vi "输入数据解析.vi"(0 "单个参数补充":dbl, 1 "从板号":dbl=1.0, 2 "主板二维码":string="BNET01", 3 "从板二维码":string="BNET01", 5 "主板引用":refnum<vi>, 7 "从板引用":refnum<vi>, 9 "主板选项":string="三级故障阀值", 11 "枚举":enum16{"主板", "从板"}(ring), 12 "快换":bool caption="快换写入") -> (4 "输出数组":dbl[][](array[numeric]), 6 "数组长度":dbl[](array[numeric]), 8 "循环次数":i32, 10 "命令":u32, 14 "名称":string[](array[string]), 15 "命令序号":u32[](array[numeric]))   [LabVIEW 2013] (continued)
                n5736 = property class="Tbl (严格)"(reference=w15118) -> ("Value"=w15116:string[][])  [unwired: 1 in, 2 out]
                n5737 = Index Array(array=w15116, index (col)=1 ("禁用的索引 (列)")) -> (element=w15120:string[])  [unwired: 1 in]
                n5738 = Array Subset(array=w15120, index=2 ("索引"), length=20.0 ("y")) -> (w15121:string[])
                n5739 = Fract/Exp String To Number(string=w15121) -> (number=w15113:dbl[])  [unwired: 4 out]
                n5740 = for {
                  N: 10 -> [_]
                  tunnel: w15113 -> [w15133]
                  tunnel: [w15124] -> w15111 mode=indexing
                  i -> [w15135]
                  w15128 = 4 ("索引")
                  n5741 = Multiply(x=w15135, y=2) -> (x*y=w15132:i32)
                  n5742 = Increment(x=w15132) -> (x+1=w15131:i32)
                  n5743 = Index Array(array=w15133, index #1=w15132, index #2=w15131) -> (element #1=w15130:dbl, element #2=w15129:dbl)
                  n5744 = call "二进制解析-8.6.vi"("索引"=w15128, "数值"=w15130) -> ("低位子数组"=w15127:i32[])  [unwired: 1 in, 2 out]
                  n5745 = call "二进制解析-8.6.vi"("索引"=w15128, "数值"=w15129) -> ("低位子数组"=w15126:i32[])  [unwired: 1 in, 2 out]
                  n5746 = Insert Into Array(array=w15127, new element=w15126) -> (w15125:i32[])  [unwired: 1 in]
                  n5747 = call "数值二进制转十进制-8.6.vi"("子数组"=w15125) -> ("十进制数值"=w15124:i32)  [unwired: 4 in]
                }
              }
            }
          }
        }
        frame "温度个数" {
          n5748 = for {
            N: 1 -> [_]
            tunnel: [w15147] -> w15141 mode=indexing
            tunnel: [w15146] -> w15140 mode=indexing
            tunnel: [w15145] -> w15139 mode=indexing
            tunnel: w15138 -> [w15144]
            i -> [w15148]
            n5749 = case shown="0, 默认" w15148 {
              tunnel: w15144 -> [w15156]
              tunnel: [w15152] -> w15147
              tunnel: [4.0 ("y")] -> w15146
              tunnel: [4 ("命令序号")] -> w15145
              frame 0, Default {
                n5750 = Unbundle By Name(w15156) -> ("项目信息 2"=w15157:refnum<vi>)
                n5751 = property class="Tbl (严格)"(reference=w15157) -> ("Value"=w15155:string[][])  [unwired: 1 in, 2 out]
                n5752 = Index Array(array=w15155, index (col)=1 ("禁用的索引 (列)")) -> (element=w15159:string[])  [unwired: 1 in]
                n5753 = Array Subset(array=w15159, index=1 ("索引"), length=1.0 ("y")) -> (w15160:string[])
                n5754 = Fract/Exp String To Number(string=w15160) -> (number=w15153:dbl[])  [unwired: 4 out]
                n5755 = for {
                  N: 1 -> [_]
                  tunnel: w15153 -> [w15171] mode=indexing
                  shift-right: [w15166] -> w15152
                  shift-left: dbl[] [] -> [w15165]
                  n5756 = Quotient & Remainder(x=w15171, y=256.0) -> (x-y*floor(x/y)=w15168:dbl, floor(x/y)=w15169:dbl)
                  n5757 = Build Array(w15169, w15168, 0.0 ("元素"), 1.0 ("元素")) -> (w15167:dbl[])
                  n5758 = Insert Into Array(array=w15165, new element=w15167) -> (w15166:dbl[])  [unwired: 1 in]
                }
              }
            }
          }
        }
        frame "加热控制参数" {
          n5759 = for {
            N: 1 -> [_]
            tunnel: w15178 -> [w15182]
            tunnel: [w15185] -> w15177 mode=indexing
            tunnel: [w15184] -> w15176 mode=indexing
            tunnel: [w15183] -> w15175 mode=indexing
            tunnel: w15174 -> [w15181]
            i -> [w15186]
            n5760 = case shown="0, 默认" w15186 {
              tunnel: w15181 -> [w15206 w15212 w15253 w15297 w15341]
              tunnel: w15182 -> [_ w15216 w15257 w15301 w15346]
              tunnel: [w15192 w15217 w15262 w15306 w15345] -> w15185
              tunnel: [7.0 w15218 w15263 w15307 w15344] -> w15184
              tunnel: [u32 5 ("命令序号") u32 2 ("命令序号") u32 3 ("命令序号") u32 4 ("命令序号") u32 1 ("命令序号")] -> w15183
              frame 0, Default {
                n5761 = Unbundle By Name(w15206) -> ("加热控制参数"=w15207:refnum<vi>)
                n5762 = property class="Clust (严格)"(reference=w15207) -> ("Value"=w15205:T5)  [unwired: 1 in, 2 out]
                n5763 = Unbundle(w15205) -> ("风机开启温度"=w15200:dbl, "风机关闭温度"=w15199:dbl, "加热开启温度"=w15196:dbl, "加热关闭温度"=w15195:dbl, "风机开启温差"=w15191:dbl, "风机关闭温差"=w15190:dbl, "加热关闭温差"=w15187:dbl)
                n5764 = call "输入分辨率计算-EV05.vi"("1字节?"=TRUE, "数值 2"=w15195, "数值"=w15196, "偏移量"=-40.0, "分辨率"=1.0) -> ("高字节 2"=w15188:dbl, "高字节1"=w15189:dbl)  [unwired: 5 out]
                n5765 = call "输入分辨率计算-EV05.vi"("1字节?"=TRUE, "数值 2"=w15199, "数值"=w15200, "偏移量"=-40.0, "分辨率"=1.0) -> ("高字节 2"=w15194:dbl, "高字节1"=w15193:dbl)  [unwired: 5 out]
                n5766 = Build Array(w15193, w15194, w15191, w15190, w15189, w15188, w15187) -> (w15192:dbl[])
              }
              frame 1 {
                # "电压起始值"
                n5767 = Unbundle By Name(w15212) -> ("项目信息 2"=w15211:refnum<vi>)
                n5768 = property class="Tbl (严格)"(reference=w15211) -> ("Value"=w15210:string[][])  [unwired: 1 in, 2 out]
                n5769 = Index Array(array=w15210, index (col)=1 ("禁用的索引 (列)")) -> (element=w15224:string[])  [unwired: 1 in]
                n5770 = Multiply(x=w15216, y=6.0) -> (x*y=w15220:dbl)
                n5771 = Divide(x=w15216, y=2.0) -> (x/y=w15214:dbl)
                n5772 = Multiply(x=w15216, y=1.5) -> (x*y=w15227:dbl)
                n5773 = Array Subset(array=w15224, index=w15220, length=w15216) -> (w15222:string[])
                n5774 = Round Toward +Infinity(x=w15214) -> (ceil(x): smallest int >= x=w15213:dbl)
                n5775 = Round Toward +Infinity(x=w15227) -> (ceil(x): smallest int >= x=w15218:dbl)
                n5776 = Fract/Exp String To Number(string=w15222) -> (number=w15225:dbl[])  [unwired: 4 out]
                n5777 = for {
                  N: w15213 -> [_]
                  tunnel: w15225 -> [w15251]
                  tunnel: [w15229] -> w15228 mode=indexing
                  i -> [w15250]
                  w15241 = 256.0 ("y")
                  n5778 = Multiply(x=w15250, y=2) -> (x*y=w15248:i32)
                  n5779 = Increment(x=w15248) -> (x+1=w15247:i32)
                  n5780 = Index Array(array=w15251, index #1=w15248, index #2=w15247) -> (element #1=w15242:dbl)  [unwired: 1 out]
                  n5781 = Quotient & Remainder(x=w15242, y=w15241) -> (x-y*floor(x/y)=w15230:dbl, floor(x/y)=w15238:dbl)
                  n5782 = Quotient & Remainder(x=w15242, y=w15241) -> (x-y*floor(x/y)=w15239:dbl, floor(x/y)=w15240:dbl)
                  n5783 = call "二进制解析-8.6.vi"("索引"=4, "数值"=w15238) -> ("低位子数组"=w15234:i32[])  [unwired: 3 out]
                  n5784 = call "二进制解析-8.6.vi"("索引"=4, "数值"=w15240) -> ("低位子数组"=w15237:i32[])  [unwired: 3 out]
                  n5785 = call "二进制解析-8.6.vi"("索引"=4, "数值"=w15239) -> ("低位子数组"=w15235:i32[], "高位子数组"=w15236:i32[])  [unwired: 2 out]
                  n5786 = Insert Into Array(array=w15237, new element=w15236) -> (w15244:i32[])  [unwired: 1 in]
                  n5787 = Insert Into Array(array=w15235, new element=w15234) -> (w15233:i32[])  [unwired: 1 in]
                  n5788 = call "数值二进制转十进制-8.6.vi"("子数组"=w15233) -> ("十进制数值"=w15231:i32)  [unwired: 4 out]
                  n5789 = call "数值二进制转十进制-8.6.vi"("子数组"=w15244) -> ("十进制数值"=w15232:i32)  [unwired: 4 out]
                  n5790 = Build Array(w15232, w15231, w15230) -> (w15229:dbl[])
                }
                n5791 = Reshape Array(w15228, w15218) -> (w15217:dbl[])
              }
              frame 2 {
                # "电压起始值"
                n5792 = Unbundle By Name(w15253) -> ("项目信息 2"=w15254:refnum<vi>)
                n5793 = property class="Tbl (严格)"(reference=w15254) -> ("Value"=w15252:string[][])  [unwired: 1 in, 2 out]
                n5794 = Multiply(x=w15257, y=5.0) -> (x*y=w15255:dbl)
                n5795 = Index Array(array=w15252, index (col)=1 ("禁用的索引 (列)")) -> (element=w15268:string[])  [unwired: 1 in]
                n5796 = Multiply(x=w15257, y=7.0) -> (x*y=w15258:dbl)
                n5797 = Divide(x=w15255, y=2.0) -> (x/y=w15260:dbl)
                n5798 = Multiply(x=w15255, y=1.5) -> (x*y=w15271:dbl)
                n5799 = Array Subset(array=w15268, index=w15258, length=w15255) -> (w15266:string[])
                n5800 = Round Toward +Infinity(x=w15260) -> (ceil(x): smallest int >= x=w15259:dbl)
                n5801 = Round Toward +Infinity(x=w15271) -> (ceil(x): smallest int >= x=w15263:dbl)
                n5802 = Fract/Exp String To Number(string=w15266) -> (number=w15269:dbl[])  [unwired: 4 out]
                n5803 = for {
                  N: w15259 -> [_]
                  tunnel: w15269 -> [w15295]
                  tunnel: [w15273] -> w15272 mode=indexing
                  i -> [w15294]
                  w15285 = 256.0 ("y")
                  n5804 = Multiply(x=w15294, y=2) -> (x*y=w15292:i32)
                  n5805 = Increment(x=w15292) -> (x+1=w15291:i32)
                  n5806 = Index Array(array=w15295, index #1=w15292, index #2=w15291) -> (element #1=w15286:dbl)  [unwired: 1 out]
                  n5807 = Quotient & Remainder(x=w15286, y=w15285) -> (x-y*floor(x/y)=w15274:dbl, floor(x/y)=w15282:dbl)
                  n5808 = Quotient & Remainder(x=w15286, y=w15285) -> (x-y*floor(x/y)=w15283:dbl, floor(x/y)=w15284:dbl)
                  n5809 = call "二进制解析-8.6.vi"("索引"=4, "数值"=w15282) -> ("低位子数组"=w15278:i32[])  [unwired: 3 out]
                  n5810 = call "二进制解析-8.6.vi"("索引"=4, "数值"=w15284) -> ("低位子数组"=w15281:i32[])  [unwired: 3 out]
                  n5811 = call "二进制解析-8.6.vi"("索引"=4, "数值"=w15283) -> ("低位子数组"=w15279:i32[], "高位子数组"=w15280:i32[])  [unwired: 2 out]
                  n5812 = Insert Into Array(array=w15281, new element=w15280) -> (w15288:i32[])  [unwired: 1 in]
                  n5813 = Insert Into Array(array=w15279, new element=w15278) -> (w15277:i32[])  [unwired: 1 in]
                  n5814 = call "数值二进制转十进制-8.6.vi"("子数组"=w15277) -> ("十进制数值"=w15275:i32)  [unwired: 4 out]
                  n5815 = call "数值二进制转十进制-8.6.vi"("子数组"=w15288) -> ("十进制数值"=w15276:i32)  [unwired: 4 out]
                  n5816 = Build Array(w15276, w15275, w15274) -> (w15273:dbl[])
                }
                n5817 = Reshape Array(w15272, w15263) -> (w15262:dbl[])
              }
              frame 3 {
                # "电压起始值"
                n5818 = Unbundle By Name(w15297) -> ("项目信息 2"=w15298:refnum<vi>)
                n5819 = property class="Tbl (严格)"(reference=w15298) -> ("Value"=w15296:string[][])  [unwired: 1 in, 2 out]
                n5820 = Multiply(x=w15301, y=2.0) -> (x*y=w15299:dbl)
                n5821 = Index Array(array=w15296, index (col)=1 ("禁用的索引 (列)")) -> (element=w15312:string[])  [unwired: 1 in]
                n5822 = Multiply(x=w15301, y=11.0) -> (x*y=w15302:dbl)
                n5823 = Divide(x=w15299, y=2.0) -> (x/y=w15304:dbl)
                n5824 = Multiply(x=w15299, y=1.5) -> (x*y=w15315:dbl)
                n5825 = Array Subset(array=w15312, index=w15302, length=w15299) -> (w15310:string[])
                n5826 = Round Toward +Infinity(x=w15304) -> (ceil(x): smallest int >= x=w15303:dbl)
                n5827 = Round Toward +Infinity(x=w15315) -> (ceil(x): smallest int >= x=w15307:dbl)
                n5828 = Fract/Exp String To Number(string=w15310) -> (number=w15313:dbl[])  [unwired: 4 out]
                n5829 = for {
                  N: w15303 -> [_]
                  tunnel: w15313 -> [w15339]
                  tunnel: [w15317] -> w15316 mode=indexing
                  i -> [w15338]
                  w15329 = 256.0 ("y")
                  n5830 = Multiply(x=w15338, y=2) -> (x*y=w15336:i32)
                  n5831 = Increment(x=w15336) -> (x+1=w15335:i32)
                  n5832 = Index Array(array=w15339, index #1=w15336, index #2=w15335) -> (element #1=w15330:dbl)  [unwired: 1 out]
                  n5833 = Quotient & Remainder(x=w15330, y=w15329) -> (x-y*floor(x/y)=w15318:dbl, floor(x/y)=w15326:dbl)
                  n5834 = Quotient & Remainder(x=w15330, y=w15329) -> (x-y*floor(x/y)=w15327:dbl, floor(x/y)=w15328:dbl)
                  n5835 = call "二进制解析-8.6.vi"("索引"=4, "数值"=w15326) -> ("低位子数组"=w15322:i32[])  [unwired: 3 out]
                  n5836 = call "二进制解析-8.6.vi"("索引"=4, "数值"=w15328) -> ("低位子数组"=w15325:i32[])  [unwired: 3 out]
                  n5837 = call "二进制解析-8.6.vi"("索引"=4, "数值"=w15327) -> ("低位子数组"=w15323:i32[], "高位子数组"=w15324:i32[])  [unwired: 2 out]
                  n5838 = Insert Into Array(array=w15325, new element=w15324) -> (w15332:i32[])  [unwired: 1 in]
                  n5839 = Insert Into Array(array=w15323, new element=w15322) -> (w15321:i32[])  [unwired: 1 in]
                  n5840 = call "数值二进制转十进制-8.6.vi"("子数组"=w15321) -> ("十进制数值"=w15319:i32)  [unwired: 4 out]
                  n5841 = call "数值二进制转十进制-8.6.vi"("子数组"=w15332) -> ("十进制数值"=w15320:i32)  [unwired: 4 out]
                  n5842 = Build Array(w15320, w15319, w15318) -> (w15317:dbl[])
                }
                n5843 = Reshape Array(w15316, w15307) -> (w15306:dbl[])
              }
              frame 4 {
                n5844 = Unbundle By Name(w15341) -> ("项目信息 2"=w15342:refnum<vi>)
                n5845 = property class="Tbl (严格)"(reference=w15342) -> ("Value"=w15340:string[][])  [unwired: 1 in, 2 out]
                n5846 = Index Array(array=w15340, index (col)=1 ("禁用的索引 (列)")) -> (element=w15347:string[])  [unwired: 1 in]
                n5847 = Multiply(x=w15346, y=6.0) -> (x*y=w15344:dbl)
                n5848 = Array Subset(array=w15347, index=0 ("索引"), length=w15344) -> (w15348:string[])
                n5849 = Fract/Exp String To Number(string=w15348) -> (number=w15345:dbl[])  [unwired: 4 out]
              }
            }
          }
        }
        frame "风机开启温度" {
          n5850 = for {
            N: 1 -> [_]
            tunnel: w15358 -> [w15362]
            tunnel: [w15365] -> w15357 mode=indexing
            tunnel: [w15364] -> w15356 mode=indexing
            tunnel: [w15363] -> w15355 mode=indexing
            tunnel: w15354 -> [w15361]
            i -> [w15366]
            n5851 = case shown="0, 默认" w15366 {
              tunnel: w15361 -> [w15381 w15387 w15428 w15472 w15516]
              tunnel: w15362 -> [_ w15391 w15432 w15476 w15521]
              tunnel: [w15368 w15392 w15437 w15481 w15520] -> w15365
              tunnel: [7.0 w15393 w15438 w15482 w15519] -> w15364
              tunnel: [u32 5 ("命令序号") u32 2 ("命令序号") u32 3 ("命令序号") u32 4 ("命令序号") u32 1 ("命令序号")] -> w15363
              frame 0, Default {
                w15367 = 255 ("高字节1")
                n5852 = Unbundle By Name(w15381) -> ("加热控制参数"=w15382:refnum<vi>)
                n5853 = property class="Clust (严格)"(reference=w15382) -> ("Value"=w15380:T5)  [unwired: 1 in, 2 out]
                n5854 = Unbundle(w15380) -> ("风机开启温度"=w15375:dbl, "风机关闭温度"=w15374:dbl, "加热开启温度"=w15371:dbl, "加热关闭温度"=w15370:dbl)  [unwired: 3 out]
                n5855 = call "输入分辨率计算-EV05.vi"("1字节?"=TRUE, "数值 2"=w15370, "数值"=w15371, "偏移量"=-40.0, "分辨率"=1.0) -> ()  [unwired: 7 out]
                n5856 = call "输入分辨率计算-EV05.vi"("1字节?"=TRUE, "数值 2"=w15374, "数值"=w15375, "偏移量"=-40.0, "分辨率"=1.0) -> ("高字节1"=w15369:dbl)  [unwired: 6 out]
                n5857 = Build Array(w15369, w15367, w15367, w15367, w15367, w15367, w15367) -> (w15368:dbl[])
              }
              frame 1 {
                # "电压起始值"
                n5858 = Unbundle By Name(w15387) -> ("项目信息 2"=w15386:refnum<vi>)
                n5859 = property class="Tbl (严格)"(reference=w15386) -> ("Value"=w15385:string[][])  [unwired: 1 in, 2 out]
                n5860 = Index Array(array=w15385, index (col)=1 ("禁用的索引 (列)")) -> (element=w15399:string[])  [unwired: 1 in]
                n5861 = Multiply(x=w15391, y=6.0) -> (x*y=w15395:dbl)
                n5862 = Divide(x=w15391, y=2.0) -> (x/y=w15389:dbl)
                n5863 = Multiply(x=w15391, y=1.5) -> (x*y=w15402:dbl)
                n5864 = Array Subset(array=w15399, index=w15395, length=w15391) -> (w15397:string[])
                n5865 = Round Toward +Infinity(x=w15389) -> (ceil(x): smallest int >= x=w15388:dbl)
                n5866 = Round Toward +Infinity(x=w15402) -> (ceil(x): smallest int >= x=w15393:dbl)
                n5867 = Fract/Exp String To Number(string=w15397) -> (number=w15400:dbl[])  [unwired: 4 out]
                n5868 = for {
                  N: w15388 -> [_]
                  tunnel: w15400 -> [w15426]
                  tunnel: [w15404] -> w15403 mode=indexing
                  i -> [w15425]
                  w15416 = 256.0 ("y")
                  n5869 = Multiply(x=w15425, y=2) -> (x*y=w15423:i32)
                  n5870 = Increment(x=w15423) -> (x+1=w15422:i32)
                  n5871 = Index Array(array=w15426, index #1=w15423, index #2=w15422) -> (element #1=w15417:dbl)  [unwired: 1 out]
                  n5872 = Quotient & Remainder(x=w15417, y=w15416) -> (x-y*floor(x/y)=w15405:dbl, floor(x/y)=w15413:dbl)
                  n5873 = Quotient & Remainder(x=w15417, y=w15416) -> (x-y*floor(x/y)=w15414:dbl, floor(x/y)=w15415:dbl)
                  n5874 = call "二进制解析-8.6.vi"("索引"=4, "数值"=w15413) -> ("低位子数组"=w15409:i32[])  [unwired: 3 out]
                  n5875 = call "二进制解析-8.6.vi"("索引"=4, "数值"=w15415) -> ("低位子数组"=w15412:i32[])  [unwired: 3 out]
                  n5876 = call "二进制解析-8.6.vi"("索引"=4, "数值"=w15414) -> ("低位子数组"=w15410:i32[], "高位子数组"=w15411:i32[])  [unwired: 2 out]
                  n5877 = Insert Into Array(array=w15412, new element=w15411) -> (w15419:i32[])  [unwired: 1 in]
                  n5878 = Insert Into Array(array=w15410, new element=w15409) -> (w15408:i32[])  [unwired: 1 in]
                  n5879 = call "数值二进制转十进制-8.6.vi"("子数组"=w15408) -> ("十进制数值"=w15406:i32)  [unwired: 4 out]
                  n5880 = call "数值二进制转十进制-8.6.vi"("子数组"=w15419) -> ("十进制数值"=w15407:i32)  [unwired: 4 out]
                  n5881 = Build Array(w15407, w15406, w15405) -> (w15404:dbl[])
                }
                n5882 = Reshape Array(w15403, w15393) -> (w15392:dbl[])
              }
              frame 2 {
                # "电压起始值"
                n5883 = Unbundle By Name(w15428) -> ("项目信息 2"=w15429:refnum<vi>)
                n5884 = property class="Tbl (严格)"(reference=w15429) -> ("Value"=w15427:string[][])  [unwired: 1 in, 2 out]
                n5885 = Multiply(x=w15432, y=5.0) -> (x*y=w15430:dbl)
                n5886 = Index Array(array=w15427, index (col)=1 ("禁用的索引 (列)")) -> (element=w15443:string[])  [unwired: 1 in]
                n5887 = Multiply(x=w15432, y=7.0) -> (x*y=w15433:dbl)
                n5888 = Divide(x=w15430, y=2.0) -> (x/y=w15435:dbl)
                n5889 = Multiply(x=w15430, y=1.5) -> (x*y=w15446:dbl)
                n5890 = Array Subset(array=w15443, index=w15433, length=w15430) -> (w15441:string[])
                n5891 = Round Toward +Infinity(x=w15435) -> (ceil(x): smallest int >= x=w15434:dbl)
                n5892 = Round Toward +Infinity(x=w15446) -> (ceil(x): smallest int >= x=w15438:dbl)
                n5893 = Fract/Exp String To Number(string=w15441) -> (number=w15444:dbl[])  [unwired: 4 out]
                n5894 = for {
                  N: w15434 -> [_]
                  tunnel: w15444 -> [w15470]
                  tunnel: [w15448] -> w15447 mode=indexing
                  i -> [w15469]
                  w15460 = 256.0 ("y")
                  n5895 = Multiply(x=w15469, y=2) -> (x*y=w15467:i32)
                  n5896 = Increment(x=w15467) -> (x+1=w15466:i32)
                  n5897 = Index Array(array=w15470, index #1=w15467, index #2=w15466) -> (element #1=w15461:dbl)  [unwired: 1 out]
                  n5898 = Quotient & Remainder(x=w15461, y=w15460) -> (x-y*floor(x/y)=w15449:dbl, floor(x/y)=w15457:dbl)
                  n5899 = Quotient & Remainder(x=w15461, y=w15460) -> (x-y*floor(x/y)=w15458:dbl, floor(x/y)=w15459:dbl)
                  n5900 = call "二进制解析-8.6.vi"("索引"=4, "数值"=w15457) -> ("低位子数组"=w15453:i32[])  [unwired: 3 out]
                  n5901 = call "二进制解析-8.6.vi"("索引"=4, "数值"=w15459) -> ("低位子数组"=w15456:i32[])  [unwired: 3 out]
                  n5902 = call "二进制解析-8.6.vi"("索引"=4, "数值"=w15458) -> ("低位子数组"=w15454:i32[], "高位子数组"=w15455:i32[])  [unwired: 2 out]
                  n5903 = Insert Into Array(array=w15456, new element=w15455) -> (w15463:i32[])  [unwired: 1 in]
                  n5904 = Insert Into Array(array=w15454, new element=w15453) -> (w15452:i32[])  [unwired: 1 in]
                  n5905 = call "数值二进制转十进制-8.6.vi"("子数组"=w15452) -> ("十进制数值"=w15450:i32)  [unwired: 4 out]
                  n5906 = call "数值二进制转十进制-8.6.vi"("子数组"=w15463) -> ("十进制数值"=w15451:i32)  [unwired: 4 out]
                  n5907 = Build Array(w15451, w15450, w15449) -> (w15448:dbl[])
                }
                n5908 = Reshape Array(w15447, w15438) -> (w15437:dbl[])
              }
              frame 3 {
                # "电压起始值"
                n5909 = Unbundle By Name(w15472) -> ("项目信息 2"=w15473:refnum<vi>)
                n5910 = property class="Tbl (严格)"(reference=w15473) -> ("Value"=w15471:string[][])  [unwired: 1 in, 2 out]
                n5911 = Multiply(x=w15476, y=2.0) -> (x*y=w15474:dbl)
                n5912 = Index Array(array=w15471, index (col)=1 ("禁用的索引 (列)")) -> (element=w15487:string[])  [unwired: 1 in]
                n5913 = Multiply(x=w15476, y=11.0) -> (x*y=w15477:dbl)
                n5914 = Divide(x=w15474, y=2.0) -> (x/y=w15479:dbl)
                n5915 = Multiply(x=w15474, y=1.5) -> (x*y=w15490:dbl)
                n5916 = Array Subset(array=w15487, index=w15477, length=w15474) -> (w15485:string[])
                n5917 = Round Toward +Infinity(x=w15479) -> (ceil(x): smallest int >= x=w15478:dbl)
                n5918 = Round Toward +Infinity(x=w15490) -> (ceil(x): smallest int >= x=w15482:dbl)
                n5919 = Fract/Exp String To Number(string=w15485) -> (number=w15488:dbl[])  [unwired: 4 out]
                n5920 = for {
                  N: w15478 -> [_]
                  tunnel: w15488 -> [w15514]
                  tunnel: [w15492] -> w15491 mode=indexing
                  i -> [w15513]
                  w15504 = 256.0 ("y")
                  n5921 = Multiply(x=w15513, y=2) -> (x*y=w15511:i32)
                  n5922 = Increment(x=w15511) -> (x+1=w15510:i32)
                  n5923 = Index Array(array=w15514, index #1=w15511, index #2=w15510) -> (element #1=w15505:dbl)  [unwired: 1 out]
                  n5924 = Quotient & Remainder(x=w15505, y=w15504) -> (x-y*floor(x/y)=w15493:dbl, floor(x/y)=w15501:dbl)
                  n5925 = Quotient & Remainder(x=w15505, y=w15504) -> (x-y*floor(x/y)=w15502:dbl, floor(x/y)=w15503:dbl)
                  n5926 = call "二进制解析-8.6.vi"("索引"=4, "数值"=w15501) -> ("低位子数组"=w15497:i32[])  [unwired: 3 out]
                  n5927 = call "二进制解析-8.6.vi"("索引"=4, "数值"=w15503) -> ("低位子数组"=w15500:i32[])  [unwired: 3 out]
                  n5928 = call "二进制解析-8.6.vi"("索引"=4, "数值"=w15502) -> ("低位子数组"=w15498:i32[], "高位子数组"=w15499:i32[])  [unwired: 2 out]
                  n5929 = Insert Into Array(array=w15500, new element=w15499) -> (w15507:i32[])  [unwired: 1 in]
                  n5930 = Insert Into Array(array=w15498, new element=w15497) -> (w15496:i32[])  [unwired: 1 in]
                  n5931 = call "数值二进制转十进制-8.6.vi"("子数组"=w15496) -> ("十进制数值"=w15494:i32)  [unwired: 4 out]
                  n5932 = call "数值二进制转十进制-8.6.vi"("子数组"=w15507) -> ("十进制数值"=w15495:i32)  [unwired: 4 out]
                  n5933 = Build Array(w15495, w15494, w15493) -> (w15492:dbl[])
                }
                n5934 = Reshape Array(w15491, w15482) -> (w15481:dbl[])
              }
              frame 4 {
                n5935 = Unbundle By Name(w15516) -> ("项目信息 2"=w15517:refnum<vi>)
                n5936 = property class="Tbl (严格)"(reference=w15517) -> ("Value"=w15515:string[][])  [unwired: 1 in, 2 out]
                n5937 = Index Array(array=w15515, index (col)=1 ("禁用的索引 (列)")) -> (element=w15522:string[])  [unwired: 1 in]
                n5938 = Multiply(x=w15521, y=6.0) -> (x*y=w15519:dbl)
                n5939 = Array Subset(array=w15522, index=0 ("索引"), length=w15519) -> (w15523:string[])
                n5940 = Fract/Exp String To Number(string=w15523) -> (number=w15520:dbl[])  [unwired: 4 out]
              }
            }
          }
        }
        frame "风机关闭温度" {
          n5941 = for {
            N: 1 -> [_]
            tunnel: w15533 -> [w15537]
            tunnel: [w15540] -> w15532 mode=indexing
            tunnel: [w15539] -> w15531 mode=indexing
            tunnel: [w15538] -> w15530 mode=indexing
            tunnel: w15529 -> [w15536]
            i -> [w15541]
            n5942 = case shown="0, 默认" w15541 {
              tunnel: w15536 -> [w15556 w15562 w15603 w15647 w15691]
              tunnel: w15537 -> [_ w15566 w15607 w15651 w15696]
              tunnel: [w15544 w15567 w15612 w15656 w15695] -> w15540
              tunnel: [7.0 w15568 w15613 w15657 w15694] -> w15539
              tunnel: [u32 5 ("命令序号") u32 2 ("命令序号") u32 3 ("命令序号") u32 4 ("命令序号") u32 1 ("命令序号")] -> w15538
              frame 0, Default {
                w15542 = 255 ("高字节1")
                n5943 = Unbundle By Name(w15556) -> ("加热控制参数"=w15557:refnum<vi>)
                n5944 = property class="Clust (严格)"(reference=w15557) -> ("Value"=w15555:T5)  [unwired: 1 in, 2 out]
                n5945 = Unbundle(w15555) -> ("风机开启温度"=w15550:dbl, "风机关闭温度"=w15549:dbl, "加热开启温度"=w15546:dbl, "加热关闭温度"=w15545:dbl)  [unwired: 3 out]
                n5946 = call "输入分辨率计算-EV05.vi"("1字节?"=TRUE, "数值 2"=w15545, "数值"=w15546, "偏移量"=-40.0, "分辨率"=1.0) -> ()  [unwired: 7 out]
                n5947 = call "输入分辨率计算-EV05.vi"("1字节?"=TRUE, "数值 2"=w15549, "数值"=w15550, "偏移量"=-40.0, "分辨率"=1.0) -> ("高字节 2"=w15543:dbl)  [unwired: 6 out]
                n5948 = Build Array(w15542, w15543, w15542, w15542, w15542, w15542, w15542) -> (w15544:dbl[])
              }
              frame 1 {
                # "电压起始值"
                n5949 = Unbundle By Name(w15562) -> ("项目信息 2"=w15561:refnum<vi>)
                n5950 = property class="Tbl (严格)"(reference=w15561) -> ("Value"=w15560:string[][])  [unwired: 1 in, 2 out]
                n5951 = Index Array(array=w15560, index (col)=1 ("禁用的索引 (列)")) -> (element=w15574:string[])  [unwired: 1 in]
                n5952 = Multiply(x=w15566, y=6.0) -> (x*y=w15570:dbl)
                n5953 = Divide(x=w15566, y=2.0) -> (x/y=w15564:dbl)
                n5954 = Multiply(x=w15566, y=1.5) -> (x*y=w15577:dbl)
                n5955 = Array Subset(array=w15574, index=w15570, length=w15566) -> (w15572:string[])
                n5956 = Round Toward +Infinity(x=w15564) -> (ceil(x): smallest int >= x=w15563:dbl)
                n5957 = Round Toward +Infinity(x=w15577) -> (ceil(x): smallest int >= x=w15568:dbl)
                n5958 = Fract/Exp String To Number(string=w15572) -> (number=w15575:dbl[])  [unwired: 4 out]
                n5959 = for {
                  N: w15563 -> [_]
                  tunnel: w15575 -> [w15601]
                  tunnel: [w15579] -> w15578 mode=indexing
                  i -> [w15600]
                  w15591 = 256.0 ("y")
                  n5960 = Multiply(x=w15600, y=2) -> (x*y=w15598:i32)
                  n5961 = Increment(x=w15598) -> (x+1=w15597:i32)
                  n5962 = Index Array(array=w15601, index #1=w15598, index #2=w15597) -> (element #1=w15592:dbl)  [unwired: 1 out]
                  n5963 = Quotient & Remainder(x=w15592, y=w15591) -> (x-y*floor(x/y)=w15580:dbl, floor(x/y)=w15588:dbl)
                  n5964 = Quotient & Remainder(x=w15592, y=w15591) -> (x-y*floor(x/y)=w15589:dbl, floor(x/y)=w15590:dbl)
                  n5965 = call "二进制解析-8.6.vi"("索引"=4, "数值"=w15588) -> ("低位子数组"=w15584:i32[])  [unwired: 3 out]
                  n5966 = call "二进制解析-8.6.vi"("索引"=4, "数值"=w15590) -> ("低位子数组"=w15587:i32[])  [unwired: 3 out]
                  n5967 = call "二进制解析-8.6.vi"("索引"=4, "数值"=w15589) -> ("低位子数组"=w15585:i32[], "高位子数组"=w15586:i32[])  [unwired: 2 out]
                  n5968 = Insert Into Array(array=w15587, new element=w15586) -> (w15594:i32[])  [unwired: 1 in]
                  n5969 = Insert Into Array(array=w15585, new element=w15584) -> (w15583:i32[])  [unwired: 1 in]
                  n5970 = call "数值二进制转十进制-8.6.vi"("子数组"=w15583) -> ("十进制数值"=w15581:i32)  [unwired: 4 out]
                  n5971 = call "数值二进制转十进制-8.6.vi"("子数组"=w15594) -> ("十进制数值"=w15582:i32)  [unwired: 4 out]
                  n5972 = Build Array(w15582, w15581, w15580) -> (w15579:dbl[])
                }
                n5973 = Reshape Array(w15578, w15568) -> (w15567:dbl[])
              }
              frame 2 {
                # "电压起始值"
                n5974 = Unbundle By Name(w15603) -> ("项目信息 2"=w15604:refnum<vi>)
                n5975 = property class="Tbl (严格)"(reference=w15604) -> ("Value"=w15602:string[][])  [unwired: 1 in, 2 out]
                n5976 = Multiply(x=w15607, y=5.0) -> (x*y=w15605:dbl)
                n5977 = Index Array(array=w15602, index (col)=1 ("禁用的索引 (列)")) -> (element=w15618:string[])  [unwired: 1 in]
                n5978 = Multiply(x=w15607, y=7.0) -> (x*y=w15608:dbl)
                n5979 = Divide(x=w15605, y=2.0) -> (x/y=w15610:dbl)
                n5980 = Multiply(x=w15605, y=1.5) -> (x*y=w15621:dbl)
                n5981 = Array Subset(array=w15618, index=w15608, length=w15605) -> (w15616:string[])
                n5982 = Round Toward +Infinity(x=w15610) -> (ceil(x): smallest int >= x=w15609:dbl)
                n5983 = Round Toward +Infinity(x=w15621) -> (ceil(x): smallest int >= x=w15613:dbl)
                n5984 = Fract/Exp String To Number(string=w15616) -> (number=w15619:dbl[])  [unwired: 4 out]
                n5985 = for {
                  N: w15609 -> [_]
                  tunnel: w15619 -> [w15645]
                  tunnel: [w15623] -> w15622 mode=indexing
                  i -> [w15644]
                  w15635 = 256.0 ("y")
                  n5986 = Multiply(x=w15644, y=2) -> (x*y=w15642:i32)
                  n5987 = Increment(x=w15642) -> (x+1=w15641:i32)
                  n5988 = Index Array(array=w15645, index #1=w15642, index #2=w15641) -> (element #1=w15636:dbl)  [unwired: 1 out]
                  n5989 = Quotient & Remainder(x=w15636, y=w15635) -> (x-y*floor(x/y)=w15624:dbl, floor(x/y)=w15632:dbl)
                  n5990 = Quotient & Remainder(x=w15636, y=w15635) -> (x-y*floor(x/y)=w15633:dbl, floor(x/y)=w15634:dbl)
                  n5991 = call "二进制解析-8.6.vi"("索引"=4, "数值"=w15632) -> ("低位子数组"=w15628:i32[])  [unwired: 3 out]
                  n5992 = call "二进制解析-8.6.vi"("索引"=4, "数值"=w15634) -> ("低位子数组"=w15631:i32[])  [unwired: 3 out]
                  n5993 = call "二进制解析-8.6.vi"("索引"=4, "数值"=w15633) -> ("低位子数组"=w15629:i32[], "高位子数组"=w15630:i32[])  [unwired: 2 out]
                  n5994 = Insert Into Array(array=w15631, new element=w15630) -> (w15638:i32[])  [unwired: 1 in]
                  n5995 = Insert Into Array(array=w15629, new element=w15628) -> (w15627:i32[])  [unwired: 1 in]
                  n5996 = call "数值二进制转十进制-8.6.vi"("子数组"=w15627) -> ("十进制数值"=w15625:i32)  [unwired: 4 out]
                  n5997 = call "数值二进制转十进制-8.6.vi"("子数组"=w15638) -> ("十进制数值"=w15626:i32)  [unwired: 4 out]
                  n5998 = Build Array(w15626, w15625, w15624) -> (w15623:dbl[])
                }
                n5999 = Reshape Array(w15622, w15613) -> (w15612:dbl[])
              }
              frame 3 {
                # "电压起始值"
                n6000 = Unbundle By Name(w15647) -> ("项目信息 2"=w15648:refnum<vi>)
                n6001 = property class="Tbl (严格)"(reference=w15648) -> ("Value"=w15646:string[][])  [unwired: 1 in, 2 out]
                n6002 = Multiply(x=w15651, y=2.0) -> (x*y=w15649:dbl)
                n6003 = Index Array(array=w15646, index (col)=1 ("禁用的索引 (列)")) -> (element=w15662:string[])  [unwired: 1 in]
                n6004 = Multiply(x=w15651, y=11.0) -> (x*y=w15652:dbl)
                n6005 = Divide(x=w15649, y=2.0) -> (x/y=w15654:dbl)
                n6006 = Multiply(x=w15649, y=1.5) -> (x*y=w15665:dbl)
                n6007 = Array Subset(array=w15662, index=w15652, length=w15649) -> (w15660:string[])
                n6008 = Round Toward +Infinity(x=w15654) -> (ceil(x): smallest int >= x=w15653:dbl)
                n6009 = Round Toward +Infinity(x=w15665) -> (ceil(x): smallest int >= x=w15657:dbl)
                n6010 = Fract/Exp String To Number(string=w15660) -> (number=w15663:dbl[])  [unwired: 4 out]
                n6011 = for {
                  N: w15653 -> [_]
                  tunnel: w15663 -> [w15689]
                  tunnel: [w15667] -> w15666 mode=indexing
                  i -> [w15688]
                  w15679 = 256.0 ("y")
                  n6012 = Multiply(x=w15688, y=2) -> (x*y=w15686:i32)
                  n6013 = Increment(x=w15686) -> (x+1=w15685:i32)
                  n6014 = Index Array(array=w15689, index #1=w15686, index #2=w15685) -> (element #1=w15680:dbl)  [unwired: 1 out]
                  n6015 = Quotient & Remainder(x=w15680, y=w15679) -> (x-y*floor(x/y)=w15668:dbl, floor(x/y)=w15676:dbl)
                  n6016 = Quotient & Remainder(x=w15680, y=w15679) -> (x-y*floor(x/y)=w15677:dbl, floor(x/y)=w15678:dbl)
                  n6017 = call "二进制解析-8.6.vi"("索引"=4, "数值"=w15676) -> ("低位子数组"=w15672:i32[])  [unwired: 3 out]
                  n6018 = call "二进制解析-8.6.vi"("索引"=4, "数值"=w15678) -> ("低位子数组"=w15675:i32[])  [unwired: 3 out]
                  n6019 = call "二进制解析-8.6.vi"("索引"=4, "数值"=w15677) -> ("低位子数组"=w15673:i32[], "高位子数组"=w15674:i32[])  [unwired: 2 out]
                  n6020 = Insert Into Array(array=w15675, new element=w15674) -> (w15682:i32[])  [unwired: 1 in]
                  n6021 = Insert Into Array(array=w15673, new element=w15672) -> (w15671:i32[])  [unwired: 1 in]
                  n6022 = call "数值二进制转十进制-8.6.vi"("子数组"=w15671) -> ("十进制数值"=w15669:i32)  [unwired: 4 out]
                  n6023 = call "数值二进制转十进制-8.6.vi"("子数组"=w15682) -> ("十进制数值"=w15670:i32)  [unwired: 4 out]
                  n6024 = Build Array(w15670, w15669, w15668) -> (w15667:dbl[])
                }
                n6025 = Reshape Array(w15666, w15657) -> (w15656:dbl[])
              }
              frame 4 {
                n6026 = Unbundle By Name(w15691) -> ("项目信息 2"=w15692:refnum<vi>)
                n6027 = property class="Tbl (严格)"(reference=w15692) -> ("Value"=w15690:string[][])  [unwired: 1 in, 2 out]
                n6028 = Index Array(array=w15690, index (col)=1 ("禁用的索引 (列)")) -> (element=w15697:string[])  [unwired: 1 in]
                n6029 = Multiply(x=w15696, y=6.0) -> (x*y=w15694:dbl)
                n6030 = Array Subset(array=w15697, index=0 ("索引"), length=w15694) -> (w15698:string[])
                n6031 = Fract/Exp String To Number(string=w15698) -> (number=w15695:dbl[])  [unwired: 4 out]
              }
            }
          }
        }
        frame "加热开启温度" {
          n6032 = for {
            N: 1 -> [_]
            tunnel: w15708 -> [w15712]
            tunnel: [w15715] -> w15707 mode=indexing
            tunnel: [w15714] -> w15706 mode=indexing
            tunnel: [w15713] -> w15705 mode=indexing
            tunnel: w15704 -> [w15711]
            i -> [w15716]
            n6033 = case shown="0, 默认" w15716 {
              tunnel: w15711 -> [w15731 w15737 w15778 w15822 w15866]
              tunnel: w15712 -> [_ w15741 w15782 w15826 w15871]
              tunnel: [w15719 w15742 w15787 w15831 w15870] -> w15715
              tunnel: [7.0 w15743 w15788 w15832 w15869] -> w15714
              tunnel: [u32 5 ("命令序号") u32 2 ("命令序号") u32 3 ("命令序号") u32 4 ("命令序号") u32 1 ("命令序号")] -> w15713
              frame 0, Default {
                w15717 = 255 ("高字节1")
                n6034 = Unbundle By Name(w15731) -> ("加热控制参数"=w15732:refnum<vi>)
                n6035 = property class="Clust (严格)"(reference=w15732) -> ("Value"=w15730:T5)  [unwired: 1 in, 2 out]
                n6036 = Unbundle(w15730) -> ("风机开启温度"=w15725:dbl, "风机关闭温度"=w15724:dbl, "加热开启温度"=w15721:dbl, "加热关闭温度"=w15720:dbl)  [unwired: 3 out]
                n6037 = call "输入分辨率计算-EV05.vi"("1字节?"=TRUE, "数值 2"=w15720, "数值"=w15721, "偏移量"=-40.0, "分辨率"=1.0) -> ("高字节1"=w15718:dbl)  [unwired: 6 out]
                n6038 = call "输入分辨率计算-EV05.vi"("1字节?"=TRUE, "数值 2"=w15724, "数值"=w15725, "偏移量"=-40.0, "分辨率"=1.0) -> ()  [unwired: 7 out]
                n6039 = Build Array(w15717, w15717, w15717, w15717, w15718, w15717, w15717) -> (w15719:dbl[])
              }
              frame 1 {
                # "电压起始值"
                n6040 = Unbundle By Name(w15737) -> ("项目信息 2"=w15736:refnum<vi>)
                n6041 = property class="Tbl (严格)"(reference=w15736) -> ("Value"=w15735:string[][])  [unwired: 1 in, 2 out]
                n6042 = Index Array(array=w15735, index (col)=1 ("禁用的索引 (列)")) -> (element=w15749:string[])  [unwired: 1 in]
                n6043 = Multiply(x=w15741, y=6.0) -> (x*y=w15745:dbl)
                n6044 = Divide(x=w15741, y=2.0) -> (x/y=w15739:dbl)
                n6045 = Multiply(x=w15741, y=1.5) -> (x*y=w15752:dbl)
                n6046 = Array Subset(array=w15749, index=w15745, length=w15741) -> (w15747:string[])
                n6047 = Round Toward +Infinity(x=w15739) -> (ceil(x): smallest int >= x=w15738:dbl)
                n6048 = Round Toward +Infinity(x=w15752) -> (ceil(x): smallest int >= x=w15743:dbl)
                n6049 = Fract/Exp String To Number(string=w15747) -> (number=w15750:dbl[])  [unwired: 4 out]
                n6050 = for {
                  N: w15738 -> [_]
                  tunnel: w15750 -> [w15776]
                  tunnel: [w15754] -> w15753 mode=indexing
                  i -> [w15775]
                  w15766 = 256.0 ("y")
                  n6051 = Multiply(x=w15775, y=2) -> (x*y=w15773:i32)
                  n6052 = Increment(x=w15773) -> (x+1=w15772:i32)
                  n6053 = Index Array(array=w15776, index #1=w15773, index #2=w15772) -> (element #1=w15767:dbl)  [unwired: 1 out]
                  n6054 = Quotient & Remainder(x=w15767, y=w15766) -> (x-y*floor(x/y)=w15755:dbl, floor(x/y)=w15763:dbl)
                  n6055 = Quotient & Remainder(x=w15767, y=w15766) -> (x-y*floor(x/y)=w15764:dbl, floor(x/y)=w15765:dbl)
                  n6056 = call "二进制解析-8.6.vi"("索引"=4, "数值"=w15763) -> ("低位子数组"=w15759:i32[])  [unwired: 3 out]
                  n6057 = call "二进制解析-8.6.vi"("索引"=4, "数值"=w15765) -> ("低位子数组"=w15762:i32[])  [unwired: 3 out]
                  n6058 = call "二进制解析-8.6.vi"("索引"=4, "数值"=w15764) -> ("低位子数组"=w15760:i32[], "高位子数组"=w15761:i32[])  [unwired: 2 out]
                  n6059 = Insert Into Array(array=w15762, new element=w15761) -> (w15769:i32[])  [unwired: 1 in]
                  n6060 = Insert Into Array(array=w15760, new element=w15759) -> (w15758:i32[])  [unwired: 1 in]
                  n6061 = call "数值二进制转十进制-8.6.vi"("子数组"=w15758) -> ("十进制数值"=w15756:i32)  [unwired: 4 out]
                  n6062 = call "数值二进制转十进制-8.6.vi"("子数组"=w15769) -> ("十进制数值"=w15757:i32)  [unwired: 4 out]
                  n6063 = Build Array(w15757, w15756, w15755) -> (w15754:dbl[])
                }
                n6064 = Reshape Array(w15753, w15743) -> (w15742:dbl[])
              }
              frame 2 {
                # "电压起始值"
                n6065 = Unbundle By Name(w15778) -> ("项目信息 2"=w15779:refnum<vi>)
                n6066 = property class="Tbl (严格)"(reference=w15779) -> ("Value"=w15777:string[][])  [unwired: 1 in, 2 out]
                n6067 = Multiply(x=w15782, y=5.0) -> (x*y=w15780:dbl)
                n6068 = Index Array(array=w15777, index (col)=1 ("禁用的索引 (列)")) -> (element=w15793:string[])  [unwired: 1 in]
                n6069 = Multiply(x=w15782, y=7.0) -> (x*y=w15783:dbl)
                n6070 = Divide(x=w15780, y=2.0) -> (x/y=w15785:dbl)
                n6071 = Multiply(x=w15780, y=1.5) -> (x*y=w15796:dbl)
                n6072 = Array Subset(array=w15793, index=w15783, length=w15780) -> (w15791:string[])
                n6073 = Round Toward +Infinity(x=w15785) -> (ceil(x): smallest int >= x=w15784:dbl)
                n6074 = Round Toward +Infinity(x=w15796) -> (ceil(x): smallest int >= x=w15788:dbl)
                n6075 = Fract/Exp String To Number(string=w15791) -> (number=w15794:dbl[])  [unwired: 4 out]
                n6076 = for {
                  N: w15784 -> [_]
                  tunnel: w15794 -> [w15820]
                  tunnel: [w15798] -> w15797 mode=indexing
                  i -> [w15819]
                  w15810 = 256.0 ("y")
                  n6077 = Multiply(x=w15819, y=2) -> (x*y=w15817:i32)
                  n6078 = Increment(x=w15817) -> (x+1=w15816:i32)
                  n6079 = Index Array(array=w15820, index #1=w15817, index #2=w15816) -> (element #1=w15811:dbl)  [unwired: 1 out]
                  n6080 = Quotient & Remainder(x=w15811, y=w15810) -> (x-y*floor(x/y)=w15799:dbl, floor(x/y)=w15807:dbl)
                  n6081 = Quotient & Remainder(x=w15811, y=w15810) -> (x-y*floor(x/y)=w15808:dbl, floor(x/y)=w15809:dbl)
                  n6082 = call "二进制解析-8.6.vi"("索引"=4, "数值"=w15807) -> ("低位子数组"=w15803:i32[])  [unwired: 3 out]
                  n6083 = call "二进制解析-8.6.vi"("索引"=4, "数值"=w15809) -> ("低位子数组"=w15806:i32[])  [unwired: 3 out]
                  n6084 = call "二进制解析-8.6.vi"("索引"=4, "数值"=w15808) -> ("低位子数组"=w15804:i32[], "高位子数组"=w15805:i32[])  [unwired: 2 out]
                  n6085 = Insert Into Array(array=w15806, new element=w15805) -> (w15813:i32[])  [unwired: 1 in]
                  n6086 = Insert Into Array(array=w15804, new element=w15803) -> (w15802:i32[])  [unwired: 1 in]
                  n6087 = call "数值二进制转十进制-8.6.vi"("子数组"=w15802) -> ("十进制数值"=w15800:i32)  [unwired: 4 out]
                  n6088 = call "数值二进制转十进制-8.6.vi"("子数组"=w15813) -> ("十进制数值"=w15801:i32)  [unwired: 4 out]
                  n6089 = Build Array(w15801, w15800, w15799) -> (w15798:dbl[])
                }
                n6090 = Reshape Array(w15797, w15788) -> (w15787:dbl[])
              }
              frame 3 {
                # "电压起始值"
                n6091 = Unbundle By Name(w15822) -> ("项目信息 2"=w15823:refnum<vi>)
                n6092 = property class="Tbl (严格)"(reference=w15823) -> ("Value"=w15821:string[][])  [unwired: 1 in, 2 out]
                n6093 = Multiply(x=w15826, y=2.0) -> (x*y=w15824:dbl)
                n6094 = Index Array(array=w15821, index (col)=1 ("禁用的索引 (列)")) -> (element=w15837:string[])  [unwired: 1 in]
                n6095 = Multiply(x=w15826, y=11.0) -> (x*y=w15827:dbl)
                n6096 = Divide(x=w15824, y=2.0) -> (x/y=w15829:dbl)
                n6097 = Multiply(x=w15824, y=1.5) -> (x*y=w15840:dbl)
                n6098 = Array Subset(array=w15837, index=w15827, length=w15824) -> (w15835:string[])
                n6099 = Round Toward +Infinity(x=w15829) -> (ceil(x): smallest int >= x=w15828:dbl)
                n6100 = Round Toward +Infinity(x=w15840) -> (ceil(x): smallest int >= x=w15832:dbl)
                n6101 = Fract/Exp String To Number(string=w15835) -> (number=w15838:dbl[])  [unwired: 4 out]
                n6102 = for {
                  N: w15828 -> [_]
                  tunnel: w15838 -> [w15864]
                  tunnel: [w15842] -> w15841 mode=indexing
                  i -> [w15863]
                  w15854 = 256.0 ("y")
                  n6103 = Multiply(x=w15863, y=2) -> (x*y=w15861:i32)
                  n6104 = Increment(x=w15861) -> (x+1=w15860:i32)
                  n6105 = Index Array(array=w15864, index #1=w15861, index #2=w15860) -> (element #1=w15855:dbl)  [unwired: 1 out]
                  n6106 = Quotient & Remainder(x=w15855, y=w15854) -> (x-y*floor(x/y)=w15843:dbl, floor(x/y)=w15851:dbl)
                  n6107 = Quotient & Remainder(x=w15855, y=w15854) -> (x-y*floor(x/y)=w15852:dbl, floor(x/y)=w15853:dbl)
                  n6108 = call "二进制解析-8.6.vi"("索引"=4, "数值"=w15851) -> ("低位子数组"=w15847:i32[])  [unwired: 3 out]
                  n6109 = call "二进制解析-8.6.vi"("索引"=4, "数值"=w15853) -> ("低位子数组"=w15850:i32[])  [unwired: 3 out]
                  n6110 = call "二进制解析-8.6.vi"("索引"=4, "数值"=w15852) -> ("低位子数组"=w15848:i32[], "高位子数组"=w15849:i32[])  [unwired: 2 out]
                  n6111 = Insert Into Array(array=w15850, new element=w15849) -> (w15857:i32[])  [unwired: 1 in]
                  n6112 = Insert Into Array(array=w15848, new element=w15847) -> (w15846:i32[])  [unwired: 1 in]
                  n6113 = call "数值二进制转十进制-8.6.vi"("子数组"=w15846) -> ("十进制数值"=w15844:i32)  [unwired: 4 out]
                  n6114 = call "数值二进制转十进制-8.6.vi"("子数组"=w15857) -> ("十进制数值"=w15845:i32)  [unwired: 4 out]
                  n6115 = Build Array(w15845, w15844, w15843) -> (w15842:dbl[])
                }
                n6116 = Reshape Array(w15841, w15832) -> (w15831:dbl[])
              }
              frame 4 {
                n6117 = Unbundle By Name(w15866) -> ("项目信息 2"=w15867:refnum<vi>)
                n6118 = property class="Tbl (严格)"(reference=w15867) -> ("Value"=w15865:string[][])  [unwired: 1 in, 2 out]
                n6119 = Index Array(array=w15865, index (col)=1 ("禁用的索引 (列)")) -> (element=w15872:string[])  [unwired: 1 in]
                n6120 = Multiply(x=w15871, y=6.0) -> (x*y=w15869:dbl)
                n6121 = Array Subset(array=w15872, index=0 ("索引"), length=w15869) -> (w15873:string[])
                n6122 = Fract/Exp String To Number(string=w15873) -> (number=w15870:dbl[])  [unwired: 4 out]
              }
            }
          }
        }
        frame "加热关闭温度" {
          n6123 = for {
            N: 1 -> [_]
            tunnel: w15883 -> [w15887]
            tunnel: [w15890] -> w15882 mode=indexing
            tunnel: [w15889] -> w15881 mode=indexing
            tunnel: [w15888] -> w15880 mode=indexing
            tunnel: w15879 -> [w15886]
            i -> [w15891]
            n6124 = case shown="0, 默认" w15891 {
              tunnel: w15886 -> [w15906 w15912 w15953 w15997 w16041]
              tunnel: w15887 -> [_ w15916 w15957 w16001 w16046]
              tunnel: [w15894 w15917 w15962 w16006 w16045] -> w15890
              tunnel: [7.0 w15918 w15963 w16007 w16044] -> w15889
              tunnel: [u32 5 ("命令序号") u32 2 ("命令序号") u32 3 ("命令序号") u32 4 ("命令序号") u32 1 ("命令序号")] -> w15888
              frame 0, Default {
                w15892 = 255 ("高字节1")
                n6125 = Unbundle By Name(w15906) -> ("加热控制参数"=w15907:refnum<vi>)
                n6126 = property class="Clust (严格)"(reference=w15907) -> ("Value"=w15905:T5)  [unwired: 1 in, 2 out]
                n6127 = Unbundle(w15905) -> ("风机开启温度"=w15900:dbl, "风机关闭温度"=w15899:dbl, "加热开启温度"=w15896:dbl, "加热关闭温度"=w15895:dbl)  [unwired: 3 out]
                n6128 = call "输入分辨率计算-EV05.vi"("1字节?"=TRUE, "数值 2"=w15895, "数值"=w15896, "偏移量"=-40.0, "分辨率"=1.0) -> ("高字节 2"=w15893:dbl)  [unwired: 6 out]
                n6129 = call "输入分辨率计算-EV05.vi"("1字节?"=TRUE, "数值 2"=w15899, "数值"=w15900, "偏移量"=-40.0, "分辨率"=1.0) -> ()  [unwired: 7 out]
                n6130 = Build Array(w15892, w15892, w15892, w15892, w15892, w15893, w15892) -> (w15894:dbl[])
              }
              frame 1 {
                # "电压起始值"
                n6131 = Unbundle By Name(w15912) -> ("项目信息 2"=w15911:refnum<vi>)
                n6132 = property class="Tbl (严格)"(reference=w15911) -> ("Value"=w15910:string[][])  [unwired: 1 in, 2 out]
                n6133 = Index Array(array=w15910, index (col)=1 ("禁用的索引 (列)")) -> (element=w15924:string[])  [unwired: 1 in]
                n6134 = Multiply(x=w15916, y=6.0) -> (x*y=w15920:dbl)
                n6135 = Divide(x=w15916, y=2.0) -> (x/y=w15914:dbl)
                n6136 = Multiply(x=w15916, y=1.5) -> (x*y=w15927:dbl)
                n6137 = Array Subset(array=w15924, index=w15920, length=w15916) -> (w15922:string[])
                n6138 = Round Toward +Infinity(x=w15914) -> (ceil(x): smallest int >= x=w15913:dbl)
                n6139 = Round Toward +Infinity(x=w15927) -> (ceil(x): smallest int >= x=w15918:dbl)
                n6140 = Fract/Exp String To Number(string=w15922) -> (number=w15925:dbl[])  [unwired: 4 out]
                n6141 = for {
                  N: w15913 -> [_]
                  tunnel: w15925 -> [w15951]
                  tunnel: [w15929] -> w15928 mode=indexing
                  i -> [w15950]
                  w15941 = 256.0 ("y")
                  n6142 = Multiply(x=w15950, y=2) -> (x*y=w15948:i32)
                  n6143 = Increment(x=w15948) -> (x+1=w15947:i32)
                  n6144 = Index Array(array=w15951, index #1=w15948, index #2=w15947) -> (element #1=w15942:dbl)  [unwired: 1 out]
                  n6145 = Quotient & Remainder(x=w15942, y=w15941) -> (x-y*floor(x/y)=w15930:dbl, floor(x/y)=w15938:dbl)
                  n6146 = Quotient & Remainder(x=w15942, y=w15941) -> (x-y*floor(x/y)=w15939:dbl, floor(x/y)=w15940:dbl)
                  n6147 = call "二进制解析-8.6.vi"("索引"=4, "数值"=w15938) -> ("低位子数组"=w15934:i32[])  [unwired: 3 out]
                  n6148 = call "二进制解析-8.6.vi"("索引"=4, "数值"=w15940) -> ("低位子数组"=w15937:i32[])  [unwired: 3 out]
                  n6149 = call "二进制解析-8.6.vi"("索引"=4, "数值"=w15939) -> ("低位子数组"=w15935:i32[], "高位子数组"=w15936:i32[])  [unwired: 2 out]
                  n6150 = Insert Into Array(array=w15937, new element=w15936) -> (w15944:i32[])  [unwired: 1 in]
                  n6151 = Insert Into Array(array=w15935, new element=w15934) -> (w15933:i32[])  [unwired: 1 in]
                  n6152 = call "数值二进制转十进制-8.6.vi"("子数组"=w15933) -> ("十进制数值"=w15931:i32)  [unwired: 4 out]
                  n6153 = call "数值二进制转十进制-8.6.vi"("子数组"=w15944) -> ("十进制数值"=w15932:i32)  [unwired: 4 out]
                  n6154 = Build Array(w15932, w15931, w15930) -> (w15929:dbl[])
                }
                n6155 = Reshape Array(w15928, w15918) -> (w15917:dbl[])
              }
              frame 2 {
                # "电压起始值"
                n6156 = Unbundle By Name(w15953) -> ("项目信息 2"=w15954:refnum<vi>)
                n6157 = property class="Tbl (严格)"(reference=w15954) -> ("Value"=w15952:string[][])  [unwired: 1 in, 2 out]
                n6158 = Multiply(x=w15957, y=5.0) -> (x*y=w15955:dbl)
                n6159 = Index Array(array=w15952, index (col)=1 ("禁用的索引 (列)")) -> (element=w15968:string[])  [unwired: 1 in]
                n6160 = Multiply(x=w15957, y=7.0) -> (x*y=w15958:dbl)
                n6161 = Divide(x=w15955, y=2.0) -> (x/y=w15960:dbl)
                n6162 = Multiply(x=w15955, y=1.5) -> (x*y=w15971:dbl)
                n6163 = Array Subset(array=w15968, index=w15958, length=w15955) -> (w15966:string[])
                n6164 = Round Toward +Infinity(x=w15960) -> (ceil(x): smallest int >= x=w15959:dbl)
                n6165 = Round Toward +Infinity(x=w15971) -> (ceil(x): smallest int >= x=w15963:dbl)
                n6166 = Fract/Exp String To Number(string=w15966) -> (number=w15969:dbl[])  [unwired: 4 out]
                n6167 = for {
                  N: w15959 -> [_]
                  tunnel: w15969 -> [w15995]
                  tunnel: [w15973] -> w15972 mode=indexing
                  i -> [w15994]
                  w15985 = 256.0 ("y")
                  n6168 = Multiply(x=w15994, y=2) -> (x*y=w15992:i32)
                  n6169 = Increment(x=w15992) -> (x+1=w15991:i32)
                  n6170 = Index Array(array=w15995, index #1=w15992, index #2=w15991) -> (element #1=w15986:dbl)  [unwired: 1 out]
                  n6171 = Quotient & Remainder(x=w15986, y=w15985) -> (x-y*floor(x/y)=w15974:dbl, floor(x/y)=w15982:dbl)
                  n6172 = Quotient & Remainder(x=w15986, y=w15985) -> (x-y*floor(x/y)=w15983:dbl, floor(x/y)=w15984:dbl)
                  n6173 = call "二进制解析-8.6.vi"("索引"=4, "数值"=w15982) -> ("低位子数组"=w15978:i32[])  [unwired: 3 out]
                  n6174 = call "二进制解析-8.6.vi"("索引"=4, "数值"=w15984) -> ("低位子数组"=w15981:i32[])  [unwired: 3 out]
                  n6175 = call "二进制解析-8.6.vi"("索引"=4, "数值"=w15983) -> ("低位子数组"=w15979:i32[], "高位子数组"=w15980:i32[])  [unwired: 2 out]
                  n6176 = Insert Into Array(array=w15981, new element=w15980) -> (w15988:i32[])  [unwired: 1 in]
                  n6177 = Insert Into Array(array=w15979, new element=w15978) -> (w15977:i32[])  [unwired: 1 in]
                  n6178 = call "数值二进制转十进制-8.6.vi"("子数组"=w15977) -> ("十进制数值"=w15975:i32)  [unwired: 4 out]
                  n6179 = call "数值二进制转十进制-8.6.vi"("子数组"=w15988) -> ("十进制数值"=w15976:i32)  [unwired: 4 out]
                  n6180 = Build Array(w15976, w15975, w15974) -> (w15973:dbl[])
                }
                n6181 = Reshape Array(w15972, w15963) -> (w15962:dbl[])
              }
              frame 3 {
                # "电压起始值"
                n6182 = Unbundle By Name(w15997) -> ("项目信息 2"=w15998:refnum<vi>)
